vi "Add.vi"(6 "Timeout":u16 format="%d ms", 8 "error in":errorcluster, 9 "Period":u16 format="%d ms", 10 "Node-ID":u8, 11 "Heartbeat in":refnum<class "Heartbeat.lvclass">) -> (0 "error out":errorcluster, 3 "Heartbeat out":refnum<class "Heartbeat.lvclass">)   [LabVIEW 2024, in "CANopen Master.lvlib" / "Heartbeat.lvclass"]
uses:
  Heartbeat.lvclass
  Heartbeat.lvclass/Heartbeat.ctl
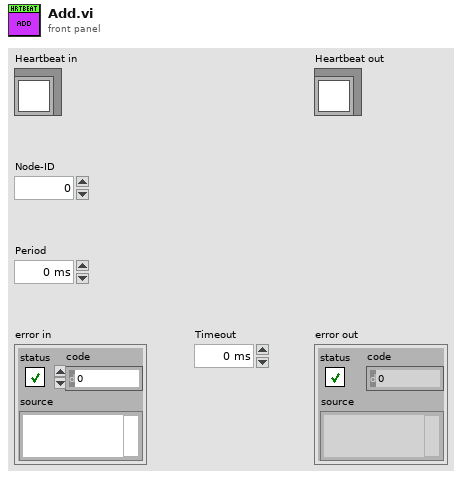
[diagram p1: front panel]
types:
  T1 = cluster{"Period":u16, "Timeout":u16, "Last Beat":timestamp}
  T2 = typedef "CANopen Master.lvlib/Heartbeat.lvclass/ObjectAttributes.ctl" = cluster{"Heartbeats":map{u8, cluster{"Period":u16, "Timeout":u16, "Last Beat":timestamp}}}
  T3 = map{u8, cluster{"Period":u16, "Timeout":u16, "Last Beat":timestamp}}
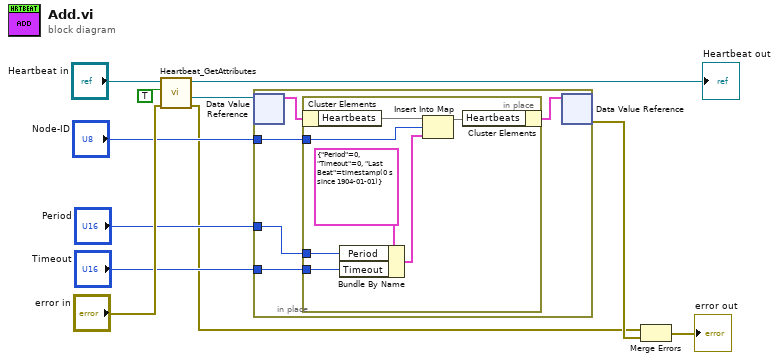
[diagram p0: block diagram]
diagram:
  n1 = call "Heartbeat_GetAttributes.vi"("Error In"="error in", "OnlyGetDvrReference(False)"=TRUE, "reference in"="Heartbeat in") -> ("Error Out"=w2:errorcluster, "DataRef"=w6:refnum<data-value>, "reference out"=→"Heartbeat out":refnum<class "Heartbeat.lvclass">)  [unwired: 5 in, 1 out]
  n2 = in-place {
    in-place-border: "Node-ID" -> [w14]
    in-place-border: "Period" -> [w13]
    in-place-border: "Timeout" -> [w12]
    n3 = in-place-dvr #1(w6) -> (w16:T2)  [unwired: 1 out]
    n4 = in-place {
      in-place-border: w14 -> [w21]
      in-place-border: w13 -> [w20]
      in-place-border: w12 -> [w19]
      n5 = in-place-cluster #2(w16) -> ("Heartbeats"=w23:T3)
      n6 = Bundle By Name(cluster=T1 {"Period"=0, "Timeout"=0, "Last Beat"=timestamp(0 s since 1904-01-01)} ("Value"), "Period"=w20, "Timeout"=w19) -> (w18:T1)
      n7 = Insert Into Map(map in=w23, key=w21, value=w18) -> (map out=w22:T3)  [unwired: 2 out]
      n8 = in-place-cluster #2("Heartbeats"=w22) -> (w15:T2)
    }
    n9 = in-place-dvr #1(w15) -> (w10:errorcluster)  [unwired: 1 out]
  }
  n10 = Merge Errors(w2, w10) -> (→"error out":errorcluster)
